vi "Self Queue Alias.vi"(11 "TEMPLATE Queue in":refnum<class "TEMPLATE Queue.lvclass">) -> (2 "Self Queue Alias":string)   [LabVIEW 2021, in "_Template.lvlib" / "Templates.lvlib" / "TEM Queue.lvlib" / "TEMPLATE Queue.lvclass"]
uses:
  TEMPLATE Queue.lvclass
  TEMPLATE Queue.lvclass/TEMPLATE Queue.ctl
  <vilib>/Nathan Davis/jettl/jettl/Queue/Queue.lvclass
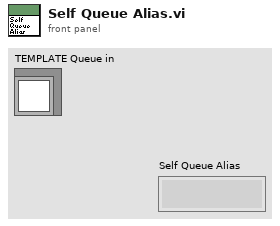
[diagram p1: front panel]
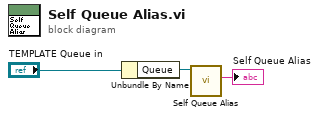
[diagram p0: block diagram]
diagram:
  n1 = Unbundle By Name("TEMPLATE Queue in") -> ("Queue"=w2:refnum<class "Queue.lvclass">)
  n2 = call-dynamic "Self Queue Alias.vi"("Queue in"=w2) -> ("Self Queue Alias"=→"Self Queue Alias":string)  [unwired: 10 in]
